vi "UI - All UI Objects Refs Memory - Typedef version.vi"(7 "Operation":T1, 8 "error in":errorcluster, 11 "VI Name (\"\" = Caller)":string) -> (0 "error out":errorcluster, 3 "Variant Out":variant)   [LabVIEW 2011]
uses:
  Controls/UI - All UI Objects Refs Memory - Operation.ctl
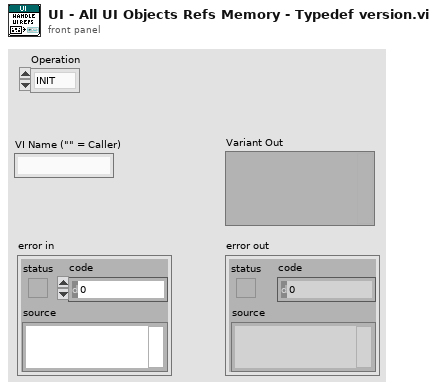
[diagram p1: front panel]
types:
  T1 = typedef "UI - All UI Objects Refs Memory - Operation.ctl" = enum16{"INIT", "GET", "ADD"}
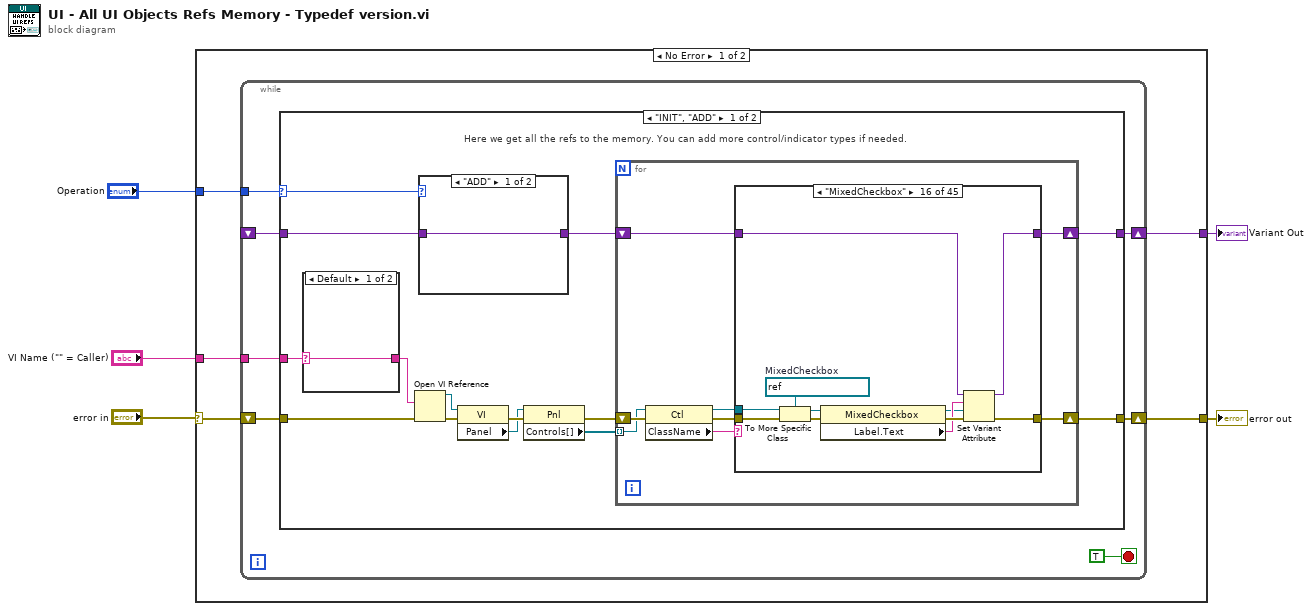
[diagram p0: block diagram]
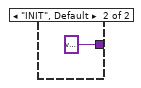
[diagram p2: hidden frame]
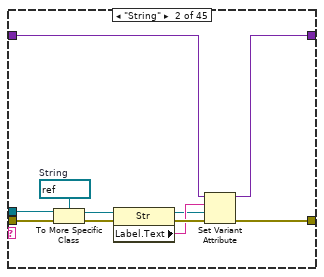
[diagram p4: hidden frame]
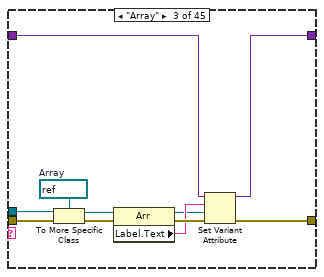
[diagram p5: hidden frame]
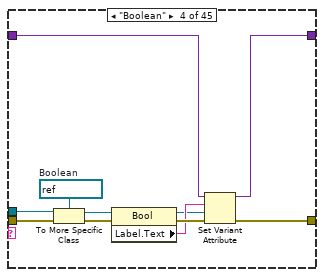
[diagram p6: hidden frame]
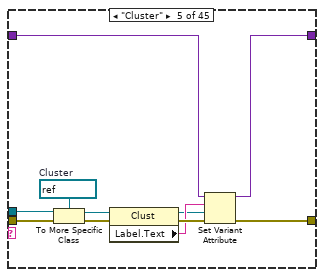
[diagram p7: hidden frame]
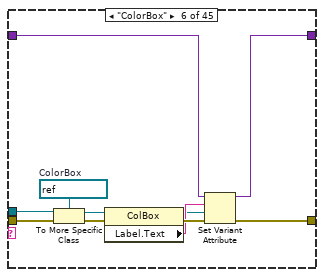
[diagram p8: hidden frame]
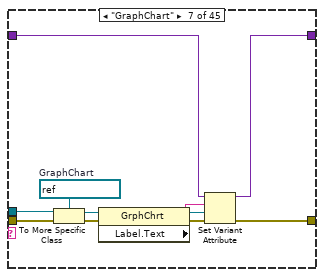
[diagram p9: hidden frame]
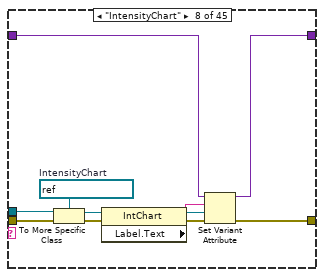
[diagram p10: hidden frame]
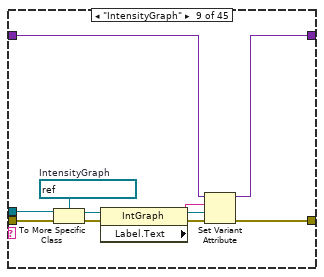
[diagram p11: hidden frame]
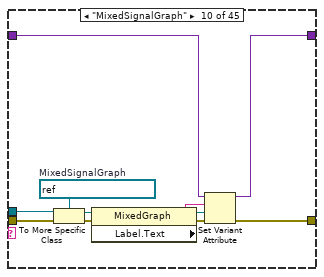
[diagram p12: hidden frame]
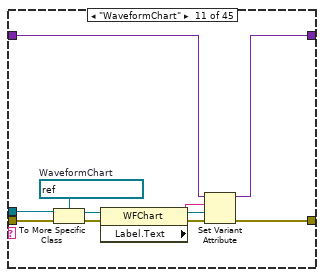
[diagram p13: hidden frame]
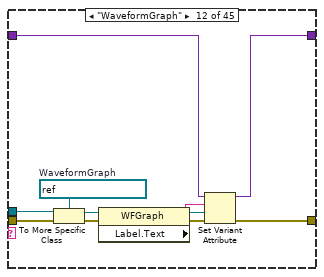
[diagram p14: hidden frame]
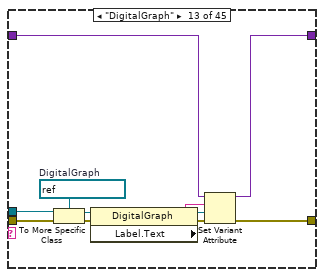
[diagram p15: hidden frame]
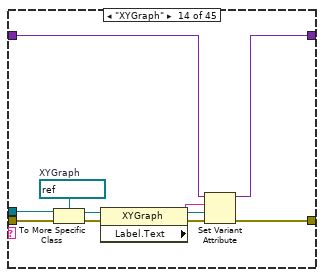
[diagram p16: hidden frame]
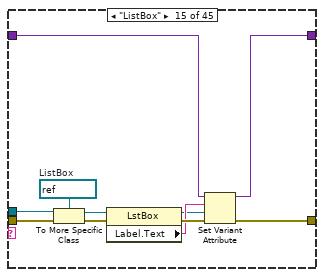
[diagram p17: hidden frame]
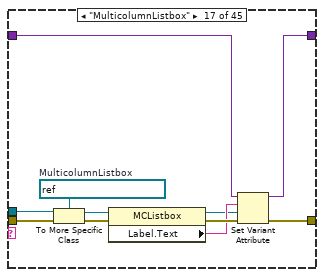
[diagram p18: hidden frame]
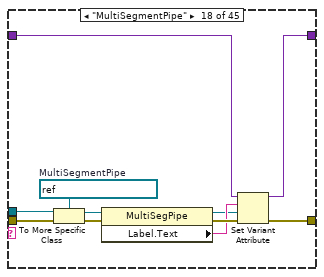
[diagram p19: hidden frame]
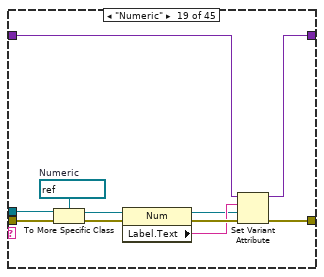
[diagram p20: hidden frame]
diagram:
  n1 = case shown="No Error" "error in" {
    selector: "error in" -> [w9 w534]
    tunnel: [w8 w534] -> w5
    tunnel: "Operation" -> [w10 _]
    tunnel: "VI Name (\"\" = Caller)" -> [w7 _]
    tunnel: [w6 _] -> w1
    frame No Error {
      n2 = while {
        tunnel: w10 -> [w16]
        shift-right: [w11] -> w8
        shift-left: w9 -> [w15]
        tunnel: w7 -> [w14]
        shift-right: [w13] -> w6
        shift-left: _ -> [w12]
        stop <- TRUE stop-if-true
        n3 = case shown="\"INIT\", \"ADD\"" w16 {
          selector: w16 -> [w20 _]
          tunnel: w15 -> [w31 w533]
          tunnel: w14 -> [w30 _]
          tunnel: [w22 w532] -> w13
          tunnel: w12 -> [w18 w532]
          tunnel: [w21 w533] -> w11
          frame "INIT", "ADD" {
            # "Here we get all the refs to the memory. You can add more control/indicator types if needed."
            n4 = case shown="Default" w30 {
              selector: w30 -> [w528 _]
              tunnel: [w528 w529] -> w29
              frame Default {
              }
              frame "" {
                # "Caller name"
                n5 = Call Chain() -> (call chain=w531:string[])
                n6 = Index Array(array=w531, index=1) -> (element=w529:string)
              }
            }
            n7 = Open VI Reference(vi path=w29, error in (no error)=w31) -> (vi reference=w27:refnum<vi>, error out=w28:errorcluster)  [unwired: 4 in]
            n8 = case shown="\"ADD\"" w20 {
              tunnel: [w32 variant] -> w19
              tunnel: w18 -> [w32 _]
              frame "ADD" {
              }
              frame "INIT", Default {
              }
            }
            n9 = property class="VI"(reference=w27, error in=w28) -> (error out=w26:errorcluster, "Panel"=w25:refnum<vi>)  [unwired: 1 out]
            n10 = property class="Pnl"(reference=w25, error in=w26) -> (error out=w23:errorcluster, "Controls[]"=w24:refnum<vi>[])  [unwired: 1 out]
            n11 = for {
              tunnel: w24 -> [w40] mode=indexing
              shift-right: [w34] -> w21
              shift-left: w23 -> [w41]
              shift-right: [w36] -> w22
              shift-left: w19 -> [w35]
              n12 = property class="Ctl"(reference=w40, error in=w41) -> (reference out=w37:refnum<vi>, error out=w39:errorcluster, "ClassName"=w38:string)
              n13 = case shown="\"MixedCheckbox\"" w38 {
                tunnel: w39 -> [w42 w54 w65 w76 w87 w98 w109 w120 w131 w142 w153 w164 w175 w186 w197 w208 w219 w230 w241 w252 w263 w274 w285 w296 w307 w318 w329 w340 w351 w362 w373 w384 w395 w406 w417 w428 w439 w450 w461 w472 w483 w494 w505 w516 w527]
                tunnel: w37 -> [_ w53 w64 w75 w86 w97 w108 w119 w130 w141 w152 w163 w174 w185 w196 w207 w218 w229 w240 w251 w262 w273 w284 w295 w306 w317 w328 w339 w350 w361 w372 w383 w394 w405 w416 w427 w438 w449 w460 w471 w482 w493 w504 w515 w526]
                tunnel: [w43 w48 w59 w70 w81 w92 w103 w114 w125 w136 w147 w158 w169 w180 w191 w202 w213 w224 w235 w246 w257 w268 w279 w290 w301 w312 w323 w334 w345 w356 w367 w378 w389 w400 w411 w422 w433 w444 w455 w466 w477 w488 w499 w510 w521] -> w36
                tunnel: w35 -> [w43 w47 w58 w69 w80 w91 w102 w113 w124 w135 w146 w157 w168 w179 w190 w201 w212 w223 w234 w245 w256 w267 w278 w289 w300 w311 w322 w333 w344 w355 w366 w377 w388 w399 w410 w421 w432 w443 w454 w465 w476 w487 w498 w509 w520]
                tunnel: [w42 w44 w55 w66 w77 w88 w99 w110 w121 w132 w143 w154 w165 w176 w187 w198 w209 w220 w231 w242 w253 w264 w275 w286 w297 w308 w319 w330 w341 w352 w363 w374 w385 w396 w407 w418 w429 w440 w451 w462 w473 w484 w495 w506 w517] -> w34
                frame Default {
                }
                frame "String" {
                  w50 = refnum<vi> refnum  # String
                  n14 = To More Specific Class(target class=w50, reference=w53, error in=w54) -> (specific class reference=w52:refnum<vi>, error out=w51:errorcluster)
                  n15 = property class="Str"(reference=w52, error in=w51) -> (reference out=w45:refnum<vi>, error out=w49:errorcluster, "Label.Text"=w46:string)
                  n16 = Set Variant Attribute(Variant=w47, name=w46, value=w45, error in=w49) -> (Variant out=w48:variant, error out=w44:errorcluster)  [unwired: 1 out]
                }
                frame "Array" {
                  w61 = refnum<vi> refnum  # Array
                  n17 = To More Specific Class(target class=w61, reference=w64, error in=w65) -> (specific class reference=w63:refnum<vi>, error out=w62:errorcluster)
                  n18 = property class="Arr"(reference=w63, error in=w62) -> (reference out=w56:refnum<vi>, error out=w60:errorcluster, "Label.Text"=w57:string)
                  n19 = Set Variant Attribute(Variant=w58, name=w57, value=w56, error in=w60) -> (Variant out=w59:variant, error out=w55:errorcluster)  [unwired: 1 out]
                }
                frame "Boolean" {
                  w72 = refnum<vi> refnum  # Boolean
                  n20 = To More Specific Class(target class=w72, reference=w75, error in=w76) -> (specific class reference=w74:refnum<vi>, error out=w73:errorcluster)
                  n21 = property class="Bool"(reference=w74, error in=w73) -> (reference out=w67:refnum<vi>, error out=w71:errorcluster, "Label.Text"=w68:string)
                  n22 = Set Variant Attribute(Variant=w69, name=w68, value=w67, error in=w71) -> (Variant out=w70:variant, error out=w66:errorcluster)  [unwired: 1 out]
                }
                frame "Cluster" {
                  w83 = refnum<vi> refnum  # Cluster
                  n23 = To More Specific Class(target class=w83, reference=w86, error in=w87) -> (specific class reference=w85:refnum<vi>, error out=w84:errorcluster)
                  n24 = property class="Clust"(reference=w85, error in=w84) -> (reference out=w78:refnum<vi>, error out=w82:errorcluster, "Label.Text"=w79:string)
                  n25 = Set Variant Attribute(Variant=w80, name=w79, value=w78, error in=w82) -> (Variant out=w81:variant, error out=w77:errorcluster)  [unwired: 1 out]
                }
                frame "ColorBox" {
                  w94 = refnum<vi> refnum  # ColorBox
                  n26 = To More Specific Class(target class=w94, reference=w97, error in=w98) -> (specific class reference=w96:refnum<vi>, error out=w95:errorcluster)
                  n27 = property class="ColBox"(reference=w96, error in=w95) -> (reference out=w89:refnum<vi>, error out=w93:errorcluster, "Label.Text"=w90:string)
                  n28 = Set Variant Attribute(Variant=w91, name=w90, value=w89, error in=w93) -> (Variant out=w92:variant, error out=w88:errorcluster)  [unwired: 1 out]
                }
                frame "GraphChart" {
                  w105 = refnum<vi> refnum  # GraphChart
                  n29 = To More Specific Class(target class=w105, reference=w108, error in=w109) -> (specific class reference=w107:refnum<vi>, error out=w106:errorcluster)
                  n30 = property class="GrphChrt"(reference=w107, error in=w106) -> (reference out=w100:refnum<vi>, error out=w104:errorcluster, "Label.Text"=w101:string)
                  n31 = Set Variant Attribute(Variant=w102, name=w101, value=w100, error in=w104) -> (Variant out=w103:variant, error out=w99:errorcluster)  [unwired: 1 out]
                }
                frame "IntensityChart" {
                  w116 = refnum<vi> refnum  # IntensityChart
                  n32 = To More Specific Class(target class=w116, reference=w119, error in=w120) -> (specific class reference=w118:refnum<vi>, error out=w117:errorcluster)
                  n33 = property class="IntChart"(reference=w118, error in=w117) -> (reference out=w111:refnum<vi>, error out=w115:errorcluster, "Label.Text"=w112:string)
                  n34 = Set Variant Attribute(Variant=w113, name=w112, value=w111, error in=w115) -> (Variant out=w114:variant, error out=w110:errorcluster)  [unwired: 1 out]
                }
                frame "IntensityGraph" {
                  w127 = refnum<vi> refnum  # IntensityGraph
                  n35 = To More Specific Class(target class=w127, reference=w130, error in=w131) -> (specific class reference=w129:refnum<vi>, error out=w128:errorcluster)
                  n36 = property class="IntGraph"(reference=w129, error in=w128) -> (reference out=w122:refnum<vi>, error out=w126:errorcluster, "Label.Text"=w123:string)
                  n37 = Set Variant Attribute(Variant=w124, name=w123, value=w122, error in=w126) -> (Variant out=w125:variant, error out=w121:errorcluster)  [unwired: 1 out]
                }
                frame "MixedSignalGraph" {
                  w138 = refnum<vi> refnum  # MixedSignalGraph
                  n38 = To More Specific Class(target class=w138, reference=w141, error in=w142) -> (specific class reference=w140:refnum<vi>, error out=w139:errorcluster)
                  n39 = property class="MixedGraph"(reference=w140, error in=w139) -> (reference out=w133:refnum<vi>, error out=w137:errorcluster, "Label.Text"=w134:string)
                  n40 = Set Variant Attribute(Variant=w135, name=w134, value=w133, error in=w137) -> (Variant out=w136:variant, error out=w132:errorcluster)  [unwired: 1 out]
                }
                frame "WaveformChart" {
                  w149 = refnum<vi> refnum  # WaveformChart
                  n41 = To More Specific Class(target class=w149, reference=w152, error in=w153) -> (specific class reference=w151:refnum<vi>, error out=w150:errorcluster)
                  n42 = property class="WFChart"(reference=w151, error in=w150) -> (reference out=w144:refnum<vi>, error out=w148:errorcluster, "Label.Text"=w145:string)
                  n43 = Set Variant Attribute(Variant=w146, name=w145, value=w144, error in=w148) -> (Variant out=w147:variant, error out=w143:errorcluster)  [unwired: 1 out]
                }
                frame "WaveformGraph" {
                  w160 = refnum<vi> refnum  # WaveformGraph
                  n44 = To More Specific Class(target class=w160, reference=w163, error in=w164) -> (specific class reference=w162:refnum<vi>, error out=w161:errorcluster)
                  n45 = property class="WFGraph"(reference=w162, error in=w161) -> (reference out=w155:refnum<vi>, error out=w159:errorcluster, "Label.Text"=w156:string)
                  n46 = Set Variant Attribute(Variant=w157, name=w156, value=w155, error in=w159) -> (Variant out=w158:variant, error out=w154:errorcluster)  [unwired: 1 out]
                }
                frame "DigitalGraph" {
                  w171 = refnum<vi> refnum  # DigitalGraph
                  n47 = To More Specific Class(target class=w171, reference=w174, error in=w175) -> (specific class reference=w173:refnum<vi>, error out=w172:errorcluster)
                  n48 = property class="DigitalGraph"(reference=w173, error in=w172) -> (reference out=w166:refnum<vi>, error out=w170:errorcluster, "Label.Text"=w167:string)
                  n49 = Set Variant Attribute(Variant=w168, name=w167, value=w166, error in=w170) -> (Variant out=w169:variant, error out=w165:errorcluster)  [unwired: 1 out]
                }
                frame "XYGraph" {
                  w182 = refnum<vi> refnum  # XYGraph
                  n50 = To More Specific Class(target class=w182, reference=w185, error in=w186) -> (specific class reference=w184:refnum<vi>, error out=w183:errorcluster)
                  n51 = property class="XYGraph"(reference=w184, error in=w183) -> (reference out=w177:refnum<vi>, error out=w181:errorcluster, "Label.Text"=w178:string)
                  n52 = Set Variant Attribute(Variant=w179, name=w178, value=w177, error in=w181) -> (Variant out=w180:variant, error out=w176:errorcluster)  [unwired: 1 out]
                }
                frame "ListBox" {
                  w193 = refnum<vi> refnum  # ListBox
                  n53 = To More Specific Class(target class=w193, reference=w196, error in=w197) -> (specific class reference=w195:refnum<vi>, error out=w194:errorcluster)
                  n54 = property class="LstBox"(reference=w195, error in=w194) -> (reference out=w188:refnum<vi>, error out=w192:errorcluster, "Label.Text"=w189:string)
                  n55 = Set Variant Attribute(Variant=w190, name=w189, value=w188, error in=w192) -> (Variant out=w191:variant, error out=w187:errorcluster)  [unwired: 1 out]
                }
                frame "MixedCheckbox" {
                  w204 = refnum<vi> refnum  # MixedCheckbox
                  n56 = To More Specific Class(target class=w204, reference=w207, error in=w208) -> (specific class reference=w206:refnum<vi>, error out=w205:errorcluster)
                  n57 = property class="MixedCheckbox"(reference=w206, error in=w205) -> (reference out=w199:refnum<vi>, error out=w203:errorcluster, "Label.Text"=w200:string)
                  n58 = Set Variant Attribute(Variant=w201, name=w200, value=w199, error in=w203) -> (Variant out=w202:variant, error out=w198:errorcluster)  [unwired: 1 out]
                }
                frame "MulticolumnListbox" {
                  w215 = refnum<vi> refnum  # MulticolumnListbox
                  n59 = To More Specific Class(target class=w215, reference=w218, error in=w219) -> (specific class reference=w217:refnum<vi>, error out=w216:errorcluster)
                  n60 = property class="MCListbox"(reference=w217, error in=w216) -> (reference out=w210:refnum<vi>, error out=w214:errorcluster, "Label.Text"=w211:string)
                  n61 = Set Variant Attribute(Variant=w212, name=w211, value=w210, error in=w214) -> (Variant out=w213:variant, error out=w209:errorcluster)  [unwired: 1 out]
                }
                frame "MultiSegmentPipe" {
                  w226 = refnum<vi> refnum  # MultiSegmentPipe
                  n62 = To More Specific Class(target class=w226, reference=w229, error in=w230) -> (specific class reference=w228:refnum<vi>, error out=w227:errorcluster)
                  n63 = property class="MultiSegPipe"(reference=w228, error in=w227) -> (reference out=w221:refnum<vi>, error out=w225:errorcluster, "Label.Text"=w222:string)
                  n64 = Set Variant Attribute(Variant=w223, name=w222, value=w221, error in=w225) -> (Variant out=w224:variant, error out=w220:errorcluster)  [unwired: 1 out]
                }
                frame "Numeric" {
                  w237 = refnum<vi> refnum  # Numeric
                  n65 = To More Specific Class(target class=w237, reference=w240, error in=w241) -> (specific class reference=w239:refnum<vi>, error out=w238:errorcluster)
                  n66 = property class="Num"(reference=w239, error in=w238) -> (reference out=w232:refnum<vi>, error out=w236:errorcluster, "Label.Text"=w233:string)
                  n67 = Set Variant Attribute(Variant=w234, name=w233, value=w232, error in=w236) -> (Variant out=w235:variant, error out=w231:errorcluster)  [unwired: 1 out]
                }
                frame "ColorRamp" {
                  w248 = refnum<vi> refnum  # ColorRamp
                  n68 = To More Specific Class(target class=w248, reference=w251, error in=w252) -> (specific class reference=w250:refnum<vi>, error out=w249:errorcluster)
                  n69 = property class="ColRmp"(reference=w250, error in=w249) -> (reference out=w243:refnum<vi>, error out=w247:errorcluster, "Label.Text"=w244:string)
                  n70 = Set Variant Attribute(Variant=w245, name=w244, value=w243, error in=w247) -> (Variant out=w246:variant, error out=w242:errorcluster)  [unwired: 1 out]
                }
                frame "Digital" {
                  w259 = refnum<vi> refnum  # Digital
                  n71 = To More Specific Class(target class=w259, reference=w262, error in=w263) -> (specific class reference=w261:refnum<vi>, error out=w260:errorcluster)
                  n72 = property class="DigNum"(reference=w261, error in=w260) -> (reference out=w254:refnum<vi>, error out=w258:errorcluster, "Label.Text"=w255:string)
                  n73 = Set Variant Attribute(Variant=w256, name=w255, value=w254, error in=w258) -> (Variant out=w257:variant, error out=w253:errorcluster)  [unwired: 1 out]
                }
                frame "NamedNumeric" {
                  w270 = refnum<vi> refnum  # NamedNumeric
                  n74 = To More Specific Class(target class=w270, reference=w273, error in=w274) -> (specific class reference=w272:refnum<vi>, error out=w271:errorcluster)
                  n75 = property class="NmdNum"(reference=w272, error in=w271) -> (reference out=w265:refnum<vi>, error out=w269:errorcluster, "Label.Text"=w266:string)
                  n76 = Set Variant Attribute(Variant=w267, name=w266, value=w265, error in=w269) -> (Variant out=w268:variant, error out=w264:errorcluster)  [unwired: 1 out]
                }
                frame "Enum" {
                  w281 = refnum<vi> refnum  # Enum
                  n77 = To More Specific Class(target class=w281, reference=w284, error in=w285) -> (specific class reference=w283:refnum<vi>, error out=w282:errorcluster)
                  n78 = property class="Enum"(reference=w283, error in=w282) -> (reference out=w276:refnum<vi>, error out=w280:errorcluster, "Label.Text"=w277:string)
                  n79 = Set Variant Attribute(Variant=w278, name=w277, value=w276, error in=w280) -> (Variant out=w279:variant, error out=w275:errorcluster)  [unwired: 1 out]
                }
                frame "Ring" {
                  w292 = refnum<vi> refnum  # Ring
                  n80 = To More Specific Class(target class=w292, reference=w295, error in=w296) -> (specific class reference=w294:refnum<vi>, error out=w293:errorcluster)
                  n81 = property class="Ring"(reference=w294, error in=w293) -> (reference out=w287:refnum<vi>, error out=w291:errorcluster, "Label.Text"=w288:string)
                  n82 = Set Variant Attribute(Variant=w289, name=w288, value=w287, error in=w291) -> (Variant out=w290:variant, error out=w286:errorcluster)  [unwired: 1 out]
                }
                frame "NumericWithScale" {
                  w303 = refnum<vi> refnum  # NumericWithScale
                  n83 = To More Specific Class(target class=w303, reference=w306, error in=w307) -> (specific class reference=w305:refnum<vi>, error out=w304:errorcluster)
                  n84 = property class="NumWthScl"(reference=w305, error in=w304) -> (reference out=w298:refnum<vi>, error out=w302:errorcluster, "Label.Text"=w299:string)
                  n85 = Set Variant Attribute(Variant=w300, name=w299, value=w298, error in=w302) -> (Variant out=w301:variant, error out=w297:errorcluster)  [unwired: 1 out]
                }
                frame "Knob" {
                  w314 = refnum<vi> refnum  # Knob
                  n86 = To More Specific Class(target class=w314, reference=w317, error in=w318) -> (specific class reference=w316:refnum<vi>, error out=w315:errorcluster)
                  n87 = property class="Knob"(reference=w316, error in=w315) -> (reference out=w309:refnum<vi>, error out=w313:errorcluster, "Label.Text"=w310:string)
                  n88 = Set Variant Attribute(Variant=w311, name=w310, value=w309, error in=w313) -> (Variant out=w312:variant, error out=w308:errorcluster)  [unwired: 1 out]
                }
                frame "Slide" {
                  w325 = refnum<vi> refnum  # Slide
                  n89 = To More Specific Class(target class=w325, reference=w328, error in=w329) -> (specific class reference=w327:refnum<vi>, error out=w326:errorcluster)
                  n90 = property class="Slide"(reference=w327, error in=w326) -> (reference out=w320:refnum<vi>, error out=w324:errorcluster, "Label.Text"=w321:string)
                  n91 = Set Variant Attribute(Variant=w322, name=w321, value=w320, error in=w324) -> (Variant out=w323:variant, error out=w319:errorcluster)  [unwired: 1 out]
                }
                frame "PageSelector" {
                  w336 = refnum<vi> refnum  # PageSelector
                  n92 = To More Specific Class(target class=w336, reference=w339, error in=w340) -> (specific class reference=w338:refnum<vi>, error out=w337:errorcluster)
                  n93 = property class="PageSel"(reference=w338, error in=w337) -> (reference out=w331:refnum<vi>, error out=w335:errorcluster, "Label.Text"=w332:string)
                  n94 = Set Variant Attribute(Variant=w333, name=w332, value=w331, error in=w335) -> (Variant out=w334:variant, error out=w330:errorcluster)  [unwired: 1 out]
                }
                frame "TabControl" {
                  w347 = refnum<vi> refnum  # TabControl
                  n95 = To More Specific Class(target class=w347, reference=w350, error in=w351) -> (specific class reference=w349:refnum<vi>, error out=w348:errorcluster)
                  n96 = property class="TabCtl"(reference=w349, error in=w348) -> (reference out=w342:refnum<vi>, error out=w346:errorcluster, "Label.Text"=w343:string)
                  n97 = Set Variant Attribute(Variant=w344, name=w343, value=w342, error in=w346) -> (Variant out=w345:variant, error out=w341:errorcluster)  [unwired: 1 out]
                }
                frame "Path" {
                  w358 = refnum<vi> refnum  # Path
                  n98 = To More Specific Class(target class=w358, reference=w361, error in=w362) -> (specific class reference=w360:refnum<vi>, error out=w359:errorcluster)
                  n99 = property class="Path"(reference=w360, error in=w359) -> (reference out=w353:refnum<vi>, error out=w357:errorcluster, "Label.Text"=w354:string)
                  n100 = Set Variant Attribute(Variant=w355, name=w354, value=w353, error in=w357) -> (Variant out=w356:variant, error out=w352:errorcluster)  [unwired: 1 out]
                }
                frame "Picture" {
                  w369 = refnum<vi> refnum  # Picture
                  n101 = To More Specific Class(target class=w369, reference=w372, error in=w373) -> (specific class reference=w371:refnum<vi>, error out=w370:errorcluster)
                  n102 = property class="Pict"(reference=w371, error in=w370) -> (reference out=w364:refnum<vi>, error out=w368:errorcluster, "Label.Text"=w365:string)
                  n103 = Set Variant Attribute(Variant=w366, name=w365, value=w364, error in=w368) -> (Variant out=w367:variant, error out=w363:errorcluster)  [unwired: 1 out]
                }
                frame "Pixmap" {
                  w380 = refnum<vi> refnum  # Pixmap
                  n104 = To More Specific Class(target class=w380, reference=w383, error in=w384) -> (specific class reference=w382:refnum<vi>, error out=w381:errorcluster)
                  n105 = property class="Pixmap"(reference=w382, error in=w381) -> (reference out=w375:refnum<vi>, error out=w379:errorcluster, "Label.Text"=w376:string)
                  n106 = Set Variant Attribute(Variant=w377, name=w376, value=w375, error in=w379) -> (Variant out=w378:variant, error out=w374:errorcluster)  [unwired: 1 out]
                }
                frame "RefNum" {
                  w391 = refnum<vi> refnum  # RefNum
                  n107 = To More Specific Class(target class=w391, reference=w394, error in=w395) -> (specific class reference=w393:refnum<vi>, error out=w392:errorcluster)
                  n108 = property class="Ref"(reference=w393, error in=w392) -> (reference out=w386:refnum<vi>, error out=w390:errorcluster, "Label.Text"=w387:string)
                  n109 = Set Variant Attribute(Variant=w388, name=w387, value=w386, error in=w390) -> (Variant out=w389:variant, error out=w385:errorcluster)  [unwired: 1 out]
                }
                frame "LVObjectRefNum" {
                  w402 = refnum<vi> refnum  # LVObjectRefNum
                  n110 = To More Specific Class(target class=w402, reference=w405, error in=w406) -> (specific class reference=w404:refnum<vi>, error out=w403:errorcluster)
                  n111 = property class="LVObjRef"(reference=w404, error in=w403) -> (reference out=w397:refnum<vi>, error out=w401:errorcluster, "Label.Text"=w398:string)
                  n112 = Set Variant Attribute(Variant=w399, name=w398, value=w397, error in=w401) -> (Variant out=w400:variant, error out=w396:errorcluster)  [unwired: 1 out]
                }
                frame "VIRefNum" {
                  w413 = refnum<vi> refnum  # VIRefNum
                  n113 = To More Specific Class(target class=w413, reference=w416, error in=w417) -> (specific class reference=w415:refnum<vi>, error out=w414:errorcluster)
                  n114 = property class="VIRef"(reference=w415, error in=w414) -> (reference out=w408:refnum<vi>, error out=w412:errorcluster, "Label.Text"=w409:string)
                  n115 = Set Variant Attribute(Variant=w410, name=w409, value=w408, error in=w412) -> (Variant out=w411:variant, error out=w407:errorcluster)  [unwired: 1 out]
                }
                frame "TypedRefNum" {
                  w424 = refnum<vi> refnum  # TypedRefNum
                  n116 = To More Specific Class(target class=w424, reference=w427, error in=w428) -> (specific class reference=w426:refnum<vi>, error out=w425:errorcluster)
                  n117 = property class="TypRef"(reference=w426, error in=w425) -> (reference out=w419:refnum<vi>, error out=w423:errorcluster, "Label.Text"=w420:string)
                  n118 = Set Variant Attribute(Variant=w421, name=w420, value=w419, error in=w423) -> (Variant out=w422:variant, error out=w418:errorcluster)  [unwired: 1 out]
                }
                frame "DataValRefNum" {
                  w435 = refnum<vi> refnum  # DataValRefNum
                  n119 = To More Specific Class(target class=w435, reference=w438, error in=w439) -> (specific class reference=w437:refnum<vi>, error out=w436:errorcluster)
                  n120 = property class="DataValRefNum"(reference=w437, error in=w436) -> (reference out=w430:refnum<vi>, error out=w434:errorcluster, "Label.Text"=w431:string)
                  n121 = Set Variant Attribute(Variant=w432, name=w431, value=w430, error in=w434) -> (Variant out=w433:variant, error out=w429:errorcluster)  [unwired: 1 out]
                }
                frame "SceneGraphDisplay" {
                  w446 = refnum<vi> refnum  # SceneGraphDisplay
                  n122 = To More Specific Class(target class=w446, reference=w449, error in=w450) -> (specific class reference=w448:refnum<vi>, error out=w447:errorcluster)
                  n123 = property class="SceneGraphDisp"(reference=w448, error in=w447) -> (reference out=w441:refnum<vi>, error out=w445:errorcluster, "Label.Text"=w442:string)
                  n124 = Set Variant Attribute(Variant=w443, name=w442, value=w441, error in=w445) -> (Variant out=w444:variant, error out=w440:errorcluster)  [unwired: 1 out]
                }
                frame "Scrollbar" {
                  w457 = refnum<vi> refnum  # Scrollbar
                  n125 = To More Specific Class(target class=w457, reference=w460, error in=w461) -> (specific class reference=w459:refnum<vi>, error out=w458:errorcluster)
                  n126 = property class="Scroll"(reference=w459, error in=w458) -> (reference out=w452:refnum<vi>, error out=w456:errorcluster, "Label.Text"=w453:string)
                  n127 = Set Variant Attribute(Variant=w454, name=w453, value=w452, error in=w456) -> (Variant out=w455:variant, error out=w451:errorcluster)  [unwired: 1 out]
                }
                frame "ComboBox" {
                  w468 = refnum<vi> refnum  # ComboBox
                  n128 = To More Specific Class(target class=w468, reference=w471, error in=w472) -> (specific class reference=w470:refnum<vi>, error out=w469:errorcluster)
                  n129 = property class="CmbBox"(reference=w470, error in=w469) -> (reference out=w463:refnum<vi>, error out=w467:errorcluster, "Label.Text"=w464:string)
                  n130 = Set Variant Attribute(Variant=w465, name=w464, value=w463, error in=w467) -> (Variant out=w466:variant, error out=w462:errorcluster)  [unwired: 1 out]
                }
                frame "SubPanel" {
                  w479 = refnum<vi> refnum  # SubPanel
                  n131 = To More Specific Class(target class=w479, reference=w482, error in=w483) -> (specific class reference=w481:refnum<vi>, error out=w480:errorcluster)
                  n132 = property class="SubPnl"(reference=w481, error in=w480) -> (reference out=w474:refnum<vi>, error out=w478:errorcluster, "Label.Text"=w475:string)
                  n133 = Set Variant Attribute(Variant=w476, name=w475, value=w474, error in=w478) -> (Variant out=w477:variant, error out=w473:errorcluster)  [unwired: 1 out]
                }
                frame "Table" {
                  w490 = refnum<vi> refnum  # Table
                  n134 = To More Specific Class(target class=w490, reference=w493, error in=w494) -> (specific class reference=w492:refnum<vi>, error out=w491:errorcluster)
                  n135 = property class="Tbl"(reference=w492, error in=w491) -> (reference out=w485:refnum<vi>, error out=w489:errorcluster, "Label.Text"=w486:string)
                  n136 = Set Variant Attribute(Variant=w487, name=w486, value=w485, error in=w489) -> (Variant out=w488:variant, error out=w484:errorcluster)  [unwired: 1 out]
                }
                frame "TreeControl" {
                  w501 = refnum<vi> refnum  # TreeControl
                  n137 = To More Specific Class(target class=w501, reference=w504, error in=w505) -> (specific class reference=w503:refnum<vi>, error out=w502:errorcluster)
                  n138 = property class="Tree"(reference=w503, error in=w502) -> (reference out=w496:refnum<vi>, error out=w500:errorcluster, "Label.Text"=w497:string)
                  n139 = Set Variant Attribute(Variant=w498, name=w497, value=w496, error in=w500) -> (Variant out=w499:variant, error out=w495:errorcluster)  [unwired: 1 out]
                }
                frame "WaveformData" {
                  w512 = refnum<vi> refnum  # WaveformData
                  n140 = To More Specific Class(target class=w512, reference=w515, error in=w516) -> (specific class reference=w514:refnum<vi>, error out=w513:errorcluster)
                  n141 = property class="WFD"(reference=w514, error in=w513) -> (reference out=w507:refnum<vi>, error out=w511:errorcluster, "Label.Text"=w508:string)
                  n142 = Set Variant Attribute(Variant=w509, name=w508, value=w507, error in=w511) -> (Variant out=w510:variant, error out=w506:errorcluster)  [unwired: 1 out]
                }
                frame "RadioButtonsControl" {
                  w523 = refnum<vi> refnum  # RadioButtonsControl
                  n143 = To More Specific Class(target class=w523, reference=w526, error in=w527) -> (specific class reference=w525:refnum<vi>, error out=w524:errorcluster)
                  n144 = property class="RadioBtnsControl"(reference=w525, error in=w524) -> (reference out=w518:refnum<vi>, error out=w522:errorcluster, "Label.Text"=w519:string)
                  n145 = Set Variant Attribute(Variant=w520, name=w519, value=w518, error in=w522) -> (Variant out=w521:variant, error out=w517:errorcluster)  [unwired: 1 out]
                }
              }
            }
          }
          frame "GET" {
            # "Here we just read out the shift register..."
          }
        }
      }
    }
    frame Error {
    }
  }
  "error out" <- w5
  "Variant Out" <- w1
